vi "Global 2.vi"() -> ()   [LabVIEW 2017]
panel:
  out "Numeric":dbl
  in  "Numeric":dbl
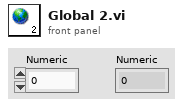
[diagram p1: front panel]
diagram:
